vi "ROI Selection.vi"() -> ()   [LabVIEW 2019, in "Algorithm.lvclass"]
uses:
  FrameworkOverrides/Algorithm.lvclass
panel:
  out "Rectangle":T1 {"Rotation" min=-90.0 max=90.0 step=1.0 format="%.2f"; "Left" scale=0.0..1024.0; "Right" scale=0.0..1024.0}
  out "error out":errorcluster
  in  "error in (no error)":errorcluster
  out "Image Out":T2(plugin-control)
  out "Reference ROI":T3 {"Contours"."Type" items=["No Selection", "Point", "Line", "Rectangle", "Oval", "Polygon", "Freehand Region", "Annulus", "Unused2", "Unused3", "Broken Line", "Freehand Line", "Rotated Rectangle"]}
  in  "File Path":path
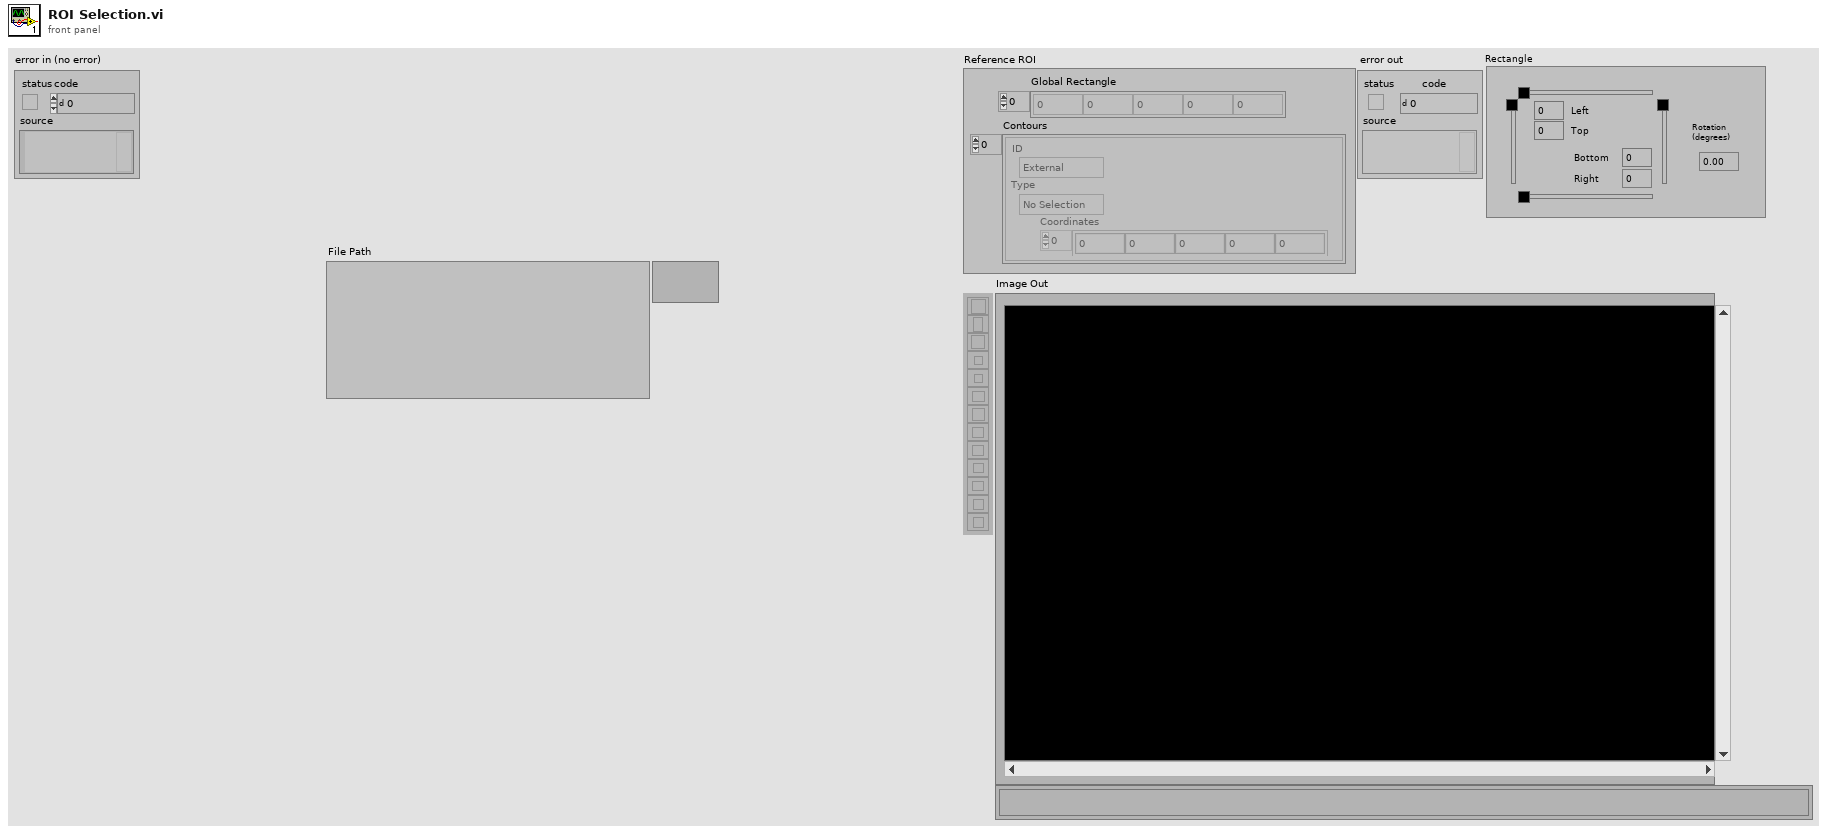
[diagram p1: front panel]
types:
  T1 = typedef "IMAQ Rectangle" = cluster{"Left":i32, "Top":i32, "Right":i32, "Bottom":i32, "Rotation":dbl}
  T2 = typedef "IMAQ Image.ctl" = refnum<image>
  T3 = typedef "ROI Descriptor" = cluster{"Global Rectangle":i32[], "Contours":cluster{"ID":enum32{"External", "Internal"}, "Type":u32, "Coordinates":i32[]}[]}
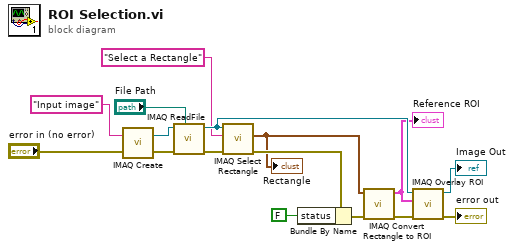
[diagram p0: block diagram]
diagram:
  n1 = call "IMAQ Create"("Image Name"="Input image", "error in (no error)"="error in (no error)") -> ("New Image"=w16:T2, "error out"=w15:errorcluster)  [unwired: 3 in]
  n2 = call "IMAQ ReadFile"("File Path"="File Path", "error in (no error)"=w15, "Image"=w16) -> ("error out"=w5:errorcluster, "Image Out"=w11:T2)  [unwired: 4 in, 3 out]
  n3 = call "IMAQ Select Rectangle"("error in (no error)"=w5, "Prompt"="Select a Rectangle", "Image In"=w11) -> ("error out"=w4:errorcluster, "Rectangle"=w1:T1)  [unwired: 5 in, 2 out]
  "Rectangle" <- w1
  n4 = Bundle By Name(cluster=w4, "status"=FALSE) -> (w2:errorcluster)
  n5 = call "IMAQ Convert Rectangle to ROI"("error in (no error)"=w2, "Rectangle"=w1) -> ("error out"=w8:errorcluster, "ROI Descriptor"=w9:T3)  [unwired: 7 in]
  "Reference ROI" <- w9
  n6 = call "IMAQ Overlay ROI"("error in (no error)"=w8, "ROI Descriptor"=w9, "Image"=w11) -> ("error out"=→"error out":errorcluster, "Image Out"=→"Image Out":T2)  [unwired: 7 in]
